vi "Reference Trajectory.vi"(6 "Trajectory Time in":dbl[](array[numeric]), 9 "Frequency":dbl, 10 "Ellipse Length":dbl[](array[numeric]), 11 "Trajectory Trigger":i32) -> (1 "Total Phase":dbl, 2 "Reference Phase":dbl, 3 "Reference X,Y":dbl[](array[numeric]), 4 "Trajectory Time out":dbl[](array[numeric]))   [LabVIEW 2021]
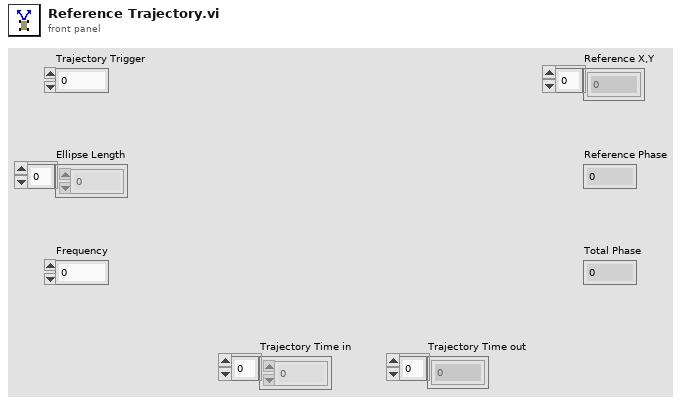
[diagram p1: front panel]
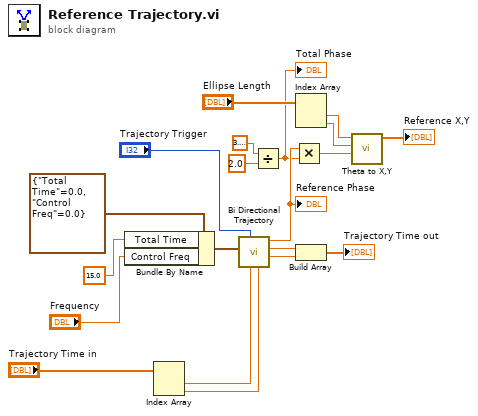
[diagram p0: block diagram]
diagram:
  n1 = Bundle By Name(cluster=cluster{"Total Time":dbl, "Control Freq":dbl} {"Total Time"=0.0, "Control Freq"=0.0} ("input cluster"), "Total Time"=15.0, "Control Freq"="Frequency") -> (w12:cluster{"Total Time":dbl, "Control Freq":dbl})
  n2 = Index Array(array="Trajectory Time in") -> (element #1=w17:dbl, element #2=w18:dbl)  [unwired: 2 in]
  n3 = call "Bi Directional Trajectory.vi"("Return Time"=w18, "Go Time"=w17, "Traj Start"="Trajectory Trigger", "Trajectory Settings"=w12) -> ("Return Next Time"=w20:dbl, "Go Next Time"=w19:dbl, "Phase"=w13:dbl)  [unwired: 5 in]
  "Reference Phase" <- w13
  n4 = Divide(x=3.141592653589793, y=2.0) -> (x/y=w2:dbl)
  "Total Phase" <- w2
  n5 = Multiply(x=w13, y=w2) -> (x*y=w14:dbl)
  n6 = Index Array(array="Ellipse Length") -> (element #1=w15:dbl, element #2=w16:dbl)  [unwired: 2 in]
  n7 = Build Array(w19, w20) -> (→"Trajectory Time out":dbl[])
  n8 = call "Theta to X,Y.vi"("theta"=w14, "b"=w16, "a"=w15) -> ("Reference X,Y"=→"Reference X,Y":dbl[])  [unwired: 8 in]
